vi "CR-字符检测参数读取1.vi"(7 "error in (no error)":errorcluster caption="错误输入（无错误）", 10 "基路径":path) -> (0 "error out":errorcluster caption="错误输出", 2 "字符识别参数":T3={"Parameters (OCR/OCV 1)"={"Threshold Data"={"Method"=enum."Local", "Looking for"=1, "Color Mode"=0, "Kernel Size"={"Width"=32, "Height"=32}, "Ranges"=[{"Min"=1, "Max"=255}]}, "Reject Border"=TRUE, "Number \nOf Erosions"=0, "Size & Spacing"={"Segment Algorithm"=0, "Min Bounding Rect Width"=1, "Max Bounding Rect Width"=65536, "Min Bounding Rect Height"=1, "Max Bounding Rect Height"=65536, "Min Character Size"=20, "Max Character Size"=65536, "Min Char Spacing"=1, "Max Horiz Element Spacing"=1, "Max Vert Element Spacing"=0, "Max Space Distance"=65536}, "Read Options"={"Read Strategy"=1, "Read Resolution"=2, "Scale Dependant"=FALSE, "Aspect Ratio"=400, "Acceptance Level"=700, "Substitution Character"="?", "MultiLine"=TRUE}, "Valid Characters"=[], "Use Text Pattern"=FALSE, "Orientation"=0, "# Lines Expected"=0, "Number of Blocks"=4}, "File Path "=path "D:/Inspect System -2/Source Code/Template Program/字符模板.abc", "Rectangle"={"Left"=0, "Top"=0, "Right"=0, "Bottom"=0, "Rotation"=0.0}, "字符长度判定"=0.0} {"Rectangle"."Rotation" min=-90.0 max=90.0 step=1.0 format="%.2f"; "Rectangle"."Left" scale=0.0..1024.0; "Rectangle"."Right" scale=0.0..1024.0; "Parameters (OCR/OCV 1)"."Threshold Data"."Looking for" items=["Light on Dark", "Dark on Light"]; "Parameters (OCR/OCV 1)"."Threshold Data"."Color Mode" items=["RGB", "HSL", "HSV", "HSI"]; "Parameters (OCR/OCV 1)"."Size & Spacing"."Segment Algorithm" items=["None", "Shortest Segment", "Legacy Auto Split"]; "Parameters (OCR/OCV 1)"."Read Options"."Read Strategy" items=["Aggressive", "Conservative"]; "Parameters (OCR/OCV 1)"."Read Options"."Read Resolution" items=["Low", "Medium", "High"]; "Parameters (OCR/OCV 1)"."Valid Characters"."Pre-defined characters" items=["Any Character", "User-defined Characters", "Alphabetic", "Alphanumeric", "Uppercase Letters", "Lowercase Letters", "Decimal Digits", "Hexadecimal Digits", "Pattern", "Force Space"]; "Parameters (OCR/OCV 1)"."Orientation" items=["Baseline inside", "Baseline outside"]}, 3 "字符检测基础参数":T1={"IsNorImage"=TRUE, "Exposure Values"=100289, "ImagePath"=path "C:/Users/hedongpo/Desktop/514-hdp/Alignment Assemble System/Test Picture/B/3.bmp"} caption="参数界面" {"Exposure Values" scale=0.0..200000.0})   [LabVIEW 2017]
uses:
  <vilib>/Utility/xml.llb/Read From XML File(string).vi
  Global System.vi
panel:
  # "UI电源线反面标签1基础参数"
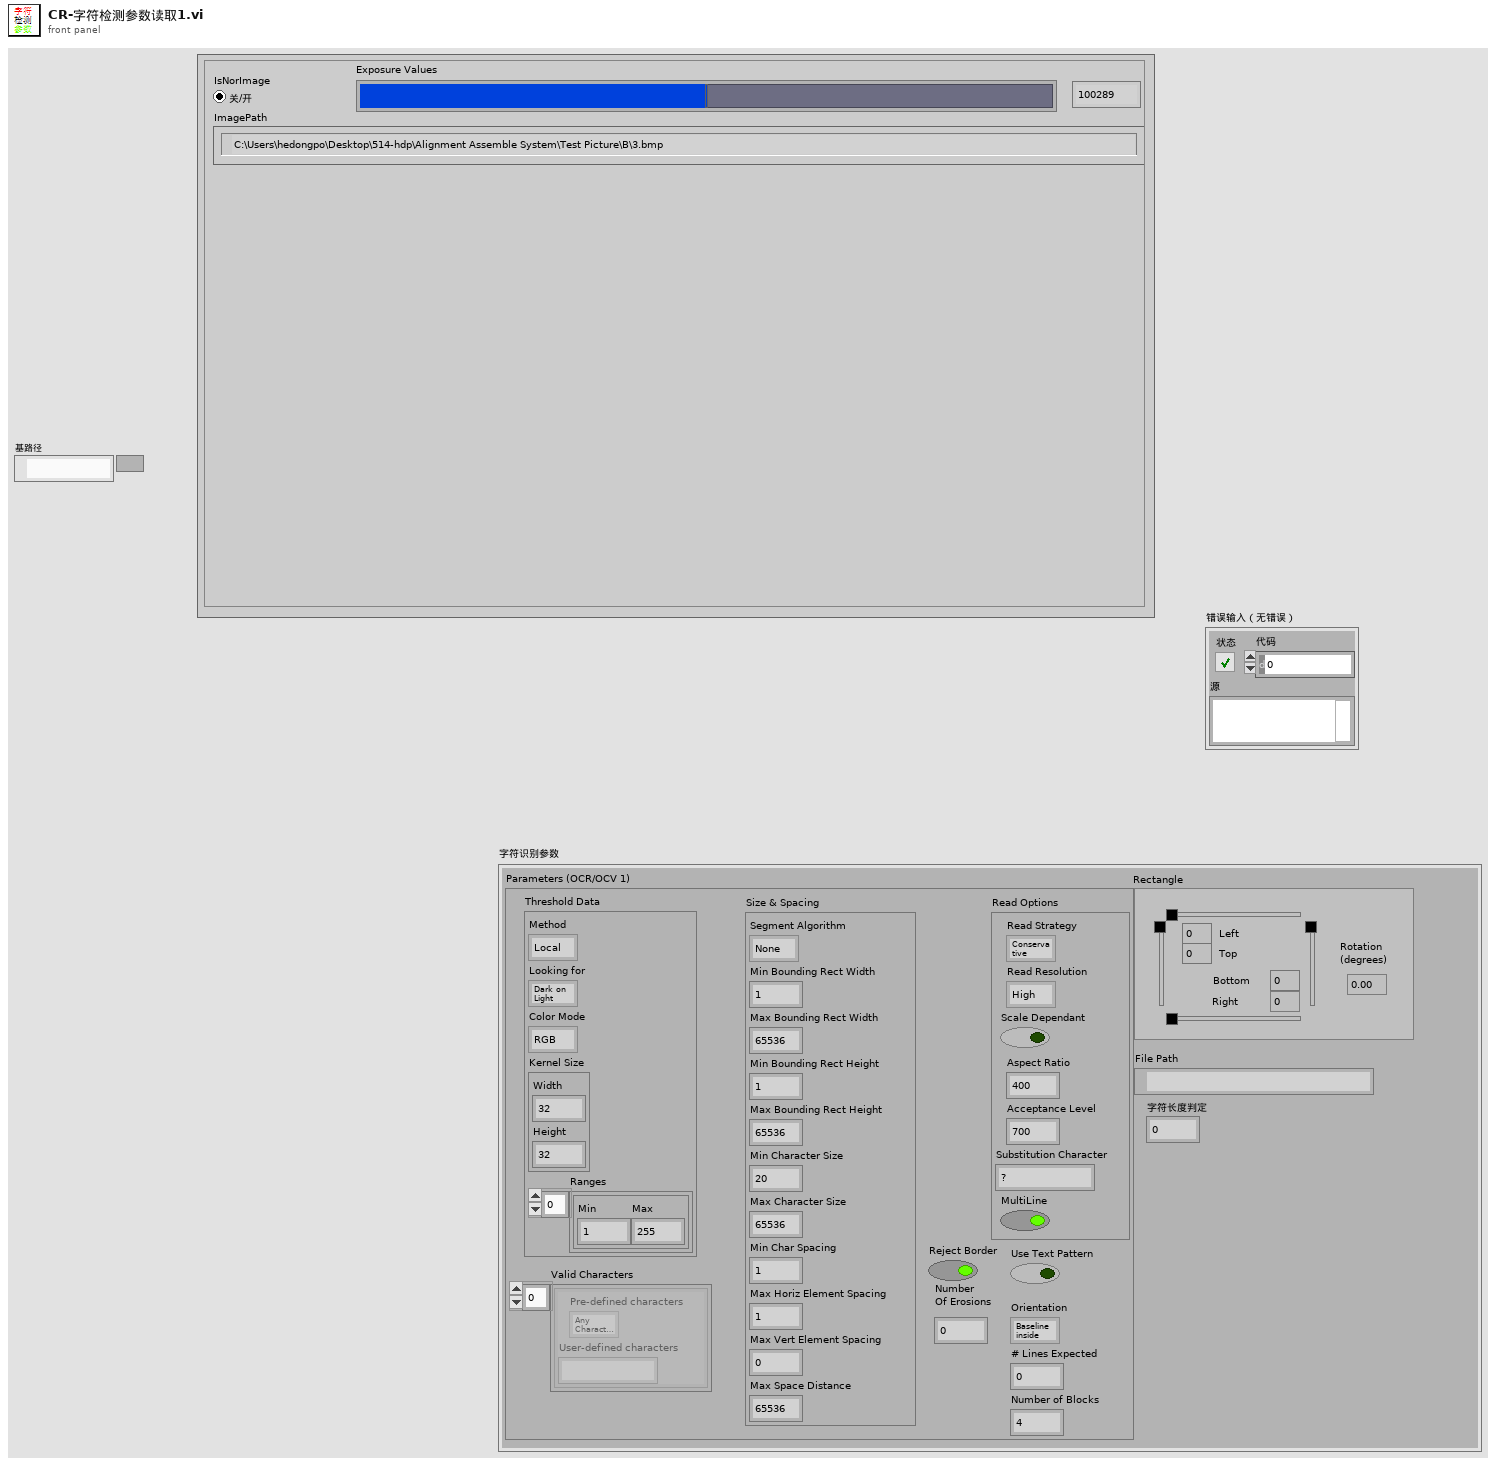
[diagram p1: front panel]
types:
  T1 = cluster{"IsNorImage":bool, "Exposure Values":u32, "ImagePath":path}
  T2 = typedef "IMAQ Rectangle" = cluster{"Left":i32, "Top":i32, "Right":i32, "Bottom":i32, "Rotation":dbl}
  T3 = cluster{"Parameters (OCR/OCV 1)":cluster{"Threshold Data":cluster{"Method":enum16{"Fixed Range", "Uniform", "Linear", "Non Linear", "Local", "Color"}, "Looking for":u32, "Color Mode":u32, "Kernel Size":cluster{"Width":i32, "Height":i32}, "Ranges":cluster{"Min":i32, "Max":i32}[]}, "Reject Border":bool, "Number \nOf Erosions":i32, "Size & Spacing":cluster{"Segment Algorithm":u16, "Min Bounding Rect Width":i32, "Max Bounding Rect Width":i32, "Min Bounding Rect Height":i32, "Max Bounding Rect Height":i32, "Min Character Size":i32, "Max Character Size":i32, "Min Char Spacing":i32, "Max Horiz Element Spacing":i32, "Max Vert Element Spacing":i32, "Max Space Distance":i32}, "Read Options":cluster{"Read Strategy":i32, "Read Resolution":i32, "Scale Dependant":bool, "Aspect Ratio":i32, "Acceptance Level":i32, "Substitution Character":string, "MultiLine":bool}, "Valid Characters":cluster{"Pre-defined characters":i32, "User-defined characters":string}[], "Use Text Pattern":bool, "Orientation":u32, "# Lines Expected":u32, "Number of Blocks":i32}, "File Path ":path, "Rectangle":T2, "字符长度判定":dbl}
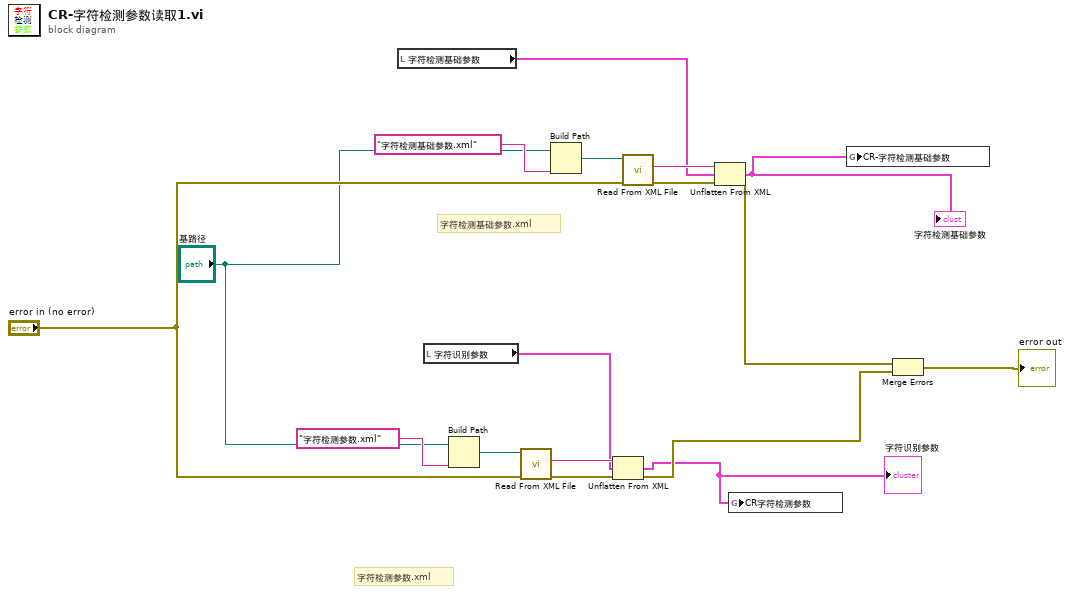
[diagram p0: block diagram]
diagram:
  # "字符检测基础参数.xml"
  # "字符检测参数.xml"
  n1 = local read "字符检测基础参数"() -> (w1:T1)
  n2 = local read "字符识别参数"() -> (w10:T3)
  n3 = Build Path(base path="基路径", name or relative path="字符检测参数.xml" ("名称或相对路径")) -> (appended path=w14:path)
  n4 = call-poly <vilib>:"Read From XML File.vi"("error in (no error)"="error in (no error)", "XML File Path"=w14) -> ("error out"=w13:errorcluster, "XML Elements"=w15:string)  [unwired: 7 in, 1 out]
  n5 = Build Path(base path="基路径", name or relative path="字符检测基础参数.xml" ("名称或相对路径")) -> (appended path=w7:path)
  n6 = Unflatten From XML(xml string=w15, type=w10, error in (no error)=w13) -> (value=w11:T3, error out=w17:errorcluster)
  "字符识别参数" <- w11
  n7 = call-poly <vilib>:"Read From XML File.vi"("error in (no error)"="error in (no error)", "XML File Path"=w7) -> ("error out"=w8:errorcluster, "XML Elements"=w6:string)  [unwired: 7 in, 1 out]
  n8 = Unflatten From XML(xml string=w6, type=w1, error in (no error)=w8) -> (value=w2:T1, error out=w4:errorcluster)
  "字符检测基础参数" <- w2
  n9 = global write "Global System.vi" "CR字符检测参数"(w11) -> ()
  n10 = global write "Global System.vi" "CR-字符检测基础参数"(w2) -> ()
  n11 = Merge Errors(w4, w17) -> (→"error out":errorcluster)
